vi "Write Limit_Regex.vi"(8 "error in (no error)":errorcluster, 10 "Limit/Regex":string, 11 "String Compare Config in":refnum<class "String Compare Config.lvclass">) -> (0 "error out":errorcluster, 3 "String Compare Config out":refnum<class "String Compare Config.lvclass">)   [LabVIEW 2015, in "String Compare Config.lvclass"]
uses:
  String Compare Config.lvclass
  String Compare Config.lvclass/String Compare Config.ctl
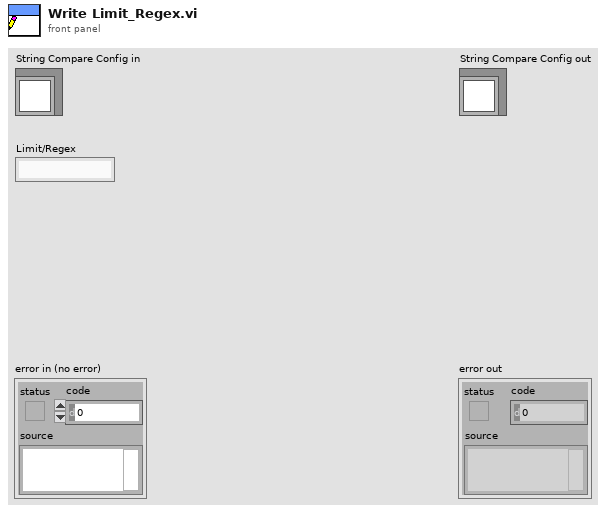
[diagram p1: front panel]
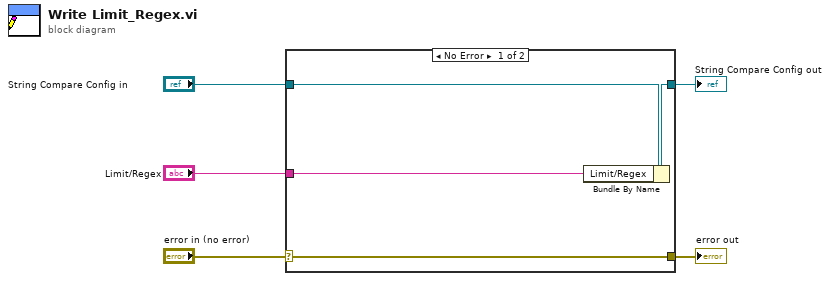
[diagram p0: block diagram]
diagram:
  n1 = case shown="No Error" "error in (no error)" {
    selector: "error in (no error)" -> [w9 w10]
    tunnel: [w9 w10] -> w4
    tunnel: [w7 w11] -> w2
    tunnel: "String Compare Config in" -> [w8 w11]
    tunnel: "Limit/Regex" -> [w6 _]
    frame No Error {
      n2 = Bundle By Name(cluster=w8, "Limit/Regex"=w6) -> (w7:refnum<class "String Compare Config.lvclass">)
    }
    frame Error {
    }
  }
  "error out" <- w4
  "String Compare Config out" <- w2
